vi "Wait for Acquisition Complete.vi"(7 "device type":T1 items=["any"=0, "AB1002"=1002, "AB1004"=1004], 8 "error in (no error)":errorcluster, 10 "Maximum Time (10000 ms)":u32=10000, 11 "VISA resource name":refnum<visa-resource-name>) -> (0 "error out":errorcluster, 3 "VISA resource name out":refnum<visa-resource-name>)   [LabVIEW 2015, in "Tausand AB1000.lvlib"]
doc: "Waits for the current acquisition to finish."
uses:
  <instrlib>/Tausand AB1000/Tausand AB1000.lvlib
  <instrlib>/Tausand AB1000/Public/Controls/deviceTypeRing.ctl
panel:
  out "maxtime reached?":bool
  out "time left ms":u32
  out "new and valid ID?":bool
  out "new ID?":bool
  out "recent ID":u32
  out "initial ID":u32
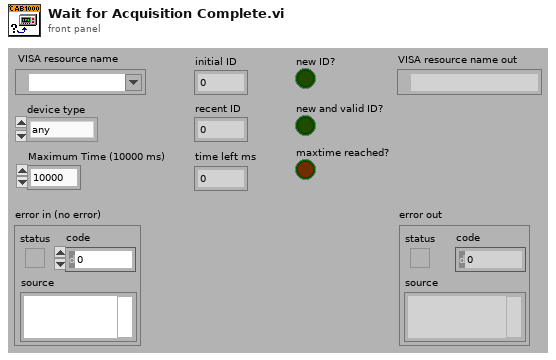
[diagram p1: front panel]
types:
  T1 = typedef "Tausand AB1000.lvlib/deviceTypeRing.ctl" = u16
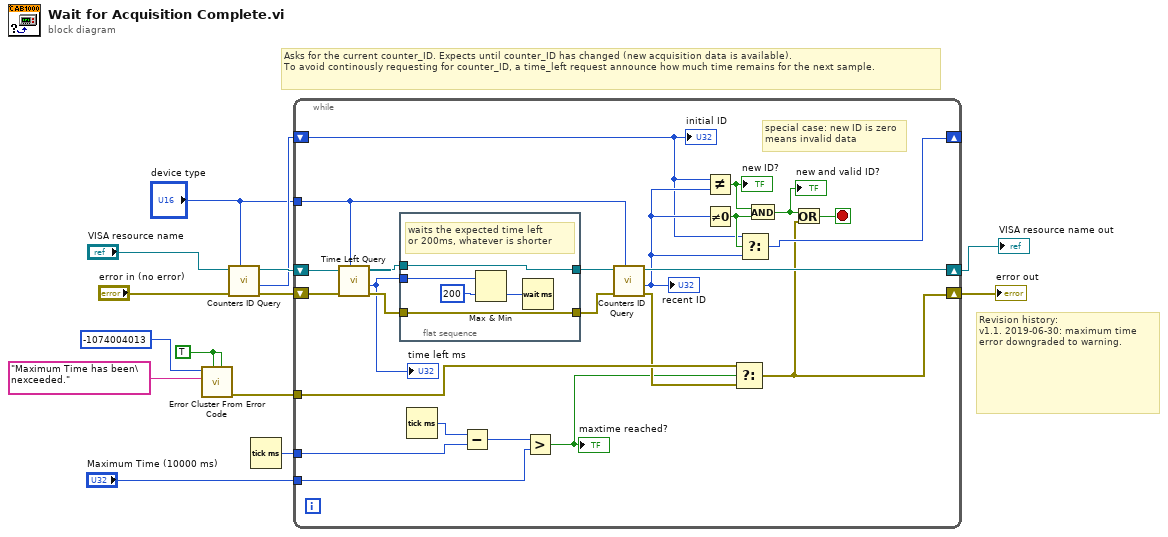
[diagram p0: block diagram]
diagram:
  w1 = TRUE ("show call chain? (False)")
  # "Revision history:\nv1.1. 2019-06-30: maximum time error downgraded to warning."
  # "Asks for the current counter_ID. Expects until counter_ID has changed (new acquisition data is available).\nTo avoid continously requesting for counter_ID, a time_left request announce how much time remains for the next sample."
  n1 = call <vilib>:"Error Cluster From Error Code.vi"("is warning? (False)"=w1, "show call chain? (False)"=w1, "error message (\"\")"="Maximum Time has been\nexceeded." ("error message (\"\")"), "error code (0)"=-1074004013) -> ("error out"=w11:errorcluster)  [unwired: 5 in]
  n2 = call <instrlib>:"Counters ID Query.vi"("device type"="device type", "error in (no error)"="error in (no error)", "VISA Refnum in"="VISA resource name") -> ("error out"=w5:errorcluster, "ID out"=w6:u32, "VISA Refnum out"=w7:refnum<visa-resource-name>)  [unwired: 5 in, 1 out]
  n3 = Tick Count (ms)() -> (millisecond timer value=w12:u32)
  n4 = while {
    tunnel: "Maximum Time (10000 ms)" -> [w35]
    tunnel: w12 -> [w36]
    tunnel: w11 -> [w34]
    shift-right: [w16] -> w4
    shift-left: w5 -> [w28]
    tunnel: "device type" -> [w17]
    shift-right: [w27] -> w3
    shift-left: w7 -> [w29]
    shift-right: [w24] -> _
    shift-left: w6 -> [w20]
    stop <- w33 stop-if-true
    # "special case: new ID is zero\nmeans invalid data"
    n5 = call <instrlib>:"Time Left Query.vi"("device type"=w17, "error in (no error)"=w28, "VISA Refnum in"=w29) -> ("error out"=w31:errorcluster, "time left ms out"=w30:u32, "VISA Refnum out"=w19:refnum<visa-resource-name>)  [unwired: 5 in, 1 out]
    "time left ms" <- w30
    n6 = flat-sequence {
      tunnel: w30 -> [w43]
      tunnel: [w40] -> w32
      tunnel: w31 -> [w40]
      tunnel: w19 -> [w39]
      tunnel: [w39] -> w18
      frame #0 {
        # "waits the expected time left \nor 200ms, whatever is shorter"
        n7 = Max & Min(x=w43, y=u32 200) -> (min(x,y)=w41:u32)  [unwired: 1 out]
        n8 = Wait (ms)(milliseconds to wait=w41) -> ()  [unwired: 1 out]
      }
    }
    n9 = Tick Count (ms)() -> (millisecond timer value=w38:u32)
    n10 = Subtract(x=w38, y=w36) -> (x-y=w37:u32)
    n11 = Greater?(x=w37, y=w35) -> (0:w15:bool)
    "maxtime reached?" <- w15
    n12 = call <instrlib>:"Counters ID Query.vi"("device type"=w17, "error in (no error)"=w32, "VISA Refnum in"=w18) -> ("error out"=w26:errorcluster, "ID out"=w25:u32, "VISA Refnum out"=w27:refnum<visa-resource-name>)  [unwired: 5 in, 1 out]
    "recent ID" <- w25
    n13 = Not Equal?(x=w20, y=w25) -> (x != y?=w23:bool)
    "new ID?" <- w23
    n14 = Not Equal To 0?(x=w25) -> (x != 0?=w22:bool)
    n15 = Select(t=w34, s=w15, f=w26) -> (s? t:f=w16:errorcluster)
    n16 = Select(t=w20, s=w22, f=w25) -> (s? t:f=w24:u32)
    n17 = And(x=w23, y=w22) -> (x .and. y?=w21:bool)
    "new and valid ID?" <- w21
    n18 = Or(x=w21, y=w16) -> (x .or. y?=w33:bool)
    "initial ID" <- w20
  }
  "error out" <- w4
  "VISA resource name out" <- w3
